vi "Wait for Acquisition Complete.vi"(8 "error in (no error)":errorcluster, 10 "Maximum Time (10000 ms)":u32=10000, 11 "VISA resource name":refnum<visa-resource-name>) -> (0 "error out":errorcluster, 3 "VISA resource name out":refnum<visa-resource-name>)   [LabVIEW 2013, in "Template - Power Meter.lvlib"]
doc: "Waits for the current acquisition to finish. This VI should be called after Initiate VI and before Fetch VI.\n\n<B>Note:</B> \n\nUse this VI only with other low-level VIs. The high-level VIs automatically incorporate this functionality. This VI does not check the instrument status."
uses:
  <instrlib>/_Template - Power Meter/Template - Power Meter.lvlib
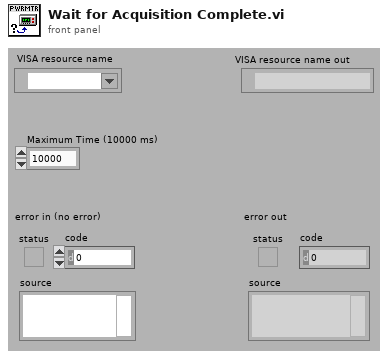
[diagram p1: front panel]
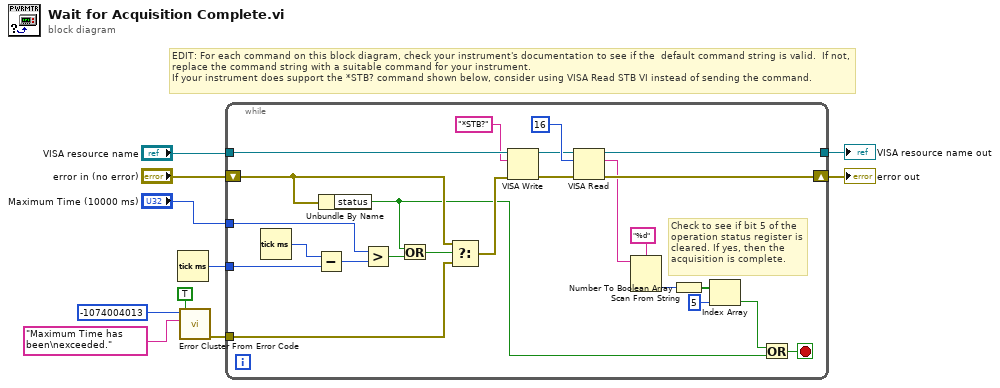
[diagram p0: block diagram]
diagram:
  # "EDIT: For each command on this block diagram, check your instrument's documentation to see if the  default command string is valid.  If not, replace the command string with a suitable command for your instrument. \nIf your instrument does support the *STB? command shown below, consider using VISA Read STB VI instead of sending the command."
  n1 = Tick Count (ms)() -> (millisecond timer value=w4:u32)
  n2 = call <vilib>:"Error Cluster From Error Code.vi"("show call chain? (False)"=TRUE, "error message (\"\")"="Maximum Time has been\nexceeded." ("error message (\"\")"), "error code (0)"=-1074004013) -> ("error out"=w3:errorcluster)  [unwired: 6 in]
  n3 = while {
    tunnel: [w33] -> w1
    tunnel: "VISA resource name" -> [w32]
    tunnel: "Maximum Time (10000 ms)" -> [w28]
    tunnel: w4 -> [w29]
    tunnel: w3 -> [w24]
    shift-right: [w34] -> w2
    shift-left: "error in (no error)" -> [w25]
    stop <- w21 stop-if-true
    # "Check to see if bit 5 of the operation status register is cleared. If yes, then the acquisition is complete."
    n4 = Tick Count (ms)() -> (millisecond timer value=w31:u32)
    n5 = Subtract(x=w31, y=w29) -> (x-y=w30:u32)
    n6 = Unbundle By Name(w25) -> ("status"=w20:bool)
    n7 = Greater?(x=w28, y=w30) -> (0:w27:bool)
    n8 = Or(x=w20, y=w27) -> (x .or. y?=w26:bool)
    n9 = Select(t=w25, s=w26, f=w24) -> (s? t:f=w23:errorcluster)
    n10 = VISA Write(VISA resource name=w32, write buffer="*STB?", error in (no error)=w23) -> (VISA resource name out=w14:refnum<visa-resource-name>, error out=w15:errorcluster)  [unwired: 1 out]
    n11 = VISA Read(VISA resource name=w14, byte count=u32 16, error in (no error)=w15) -> (VISA resource name out=w33:refnum<visa-resource-name>, read buffer=w19:string, error out=w34:errorcluster)  [unwired: 1 out]
    n12 = Scan From String(format string="%d", input string=w19) -> (output 1=w11:i32)  [unwired: 3 in, 3 out]
    n13 = Number To Boolean Array(number=w11) -> (Boolean array=w13:bool[])
    n14 = Index Array(array=w13, index=5) -> (element=w22:bool)
    n15 = Or(x=w22, y=w20) -> (x .or. y?=w21:bool)
  }
  "error out" <- w2
  "VISA resource name out" <- w1
